vi "Create Virtual Drive.vi"(8 "error in (no error)":errorcluster, 11 "BuildWorker Controller in":refnum<class "BuildWorker Controller.lvclass">) -> (0 "error out":errorcluster, 3 "BuildWorker Controller out":refnum<class "BuildWorker Controller.lvclass">)   [LabVIEW 2017, in "BuildWorker Controller.lvlib" / "BuildWorker Controller.lvclass"]
uses:
  BuildWorker Controller.lvclass
  BuildWorker Controller.lvclass/BuildWorker Controller.ctl
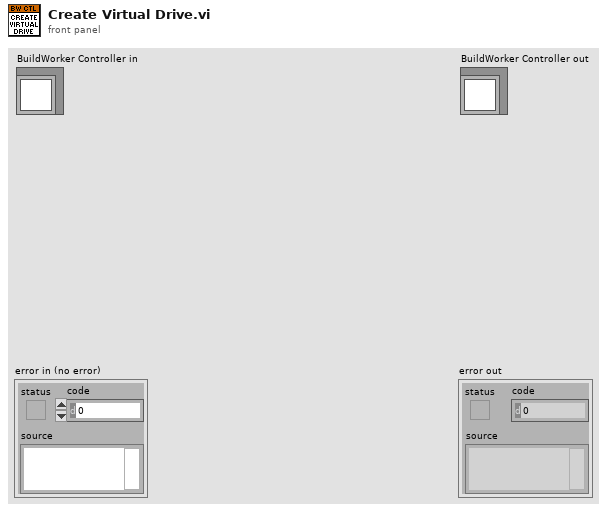
[diagram p1: front panel]
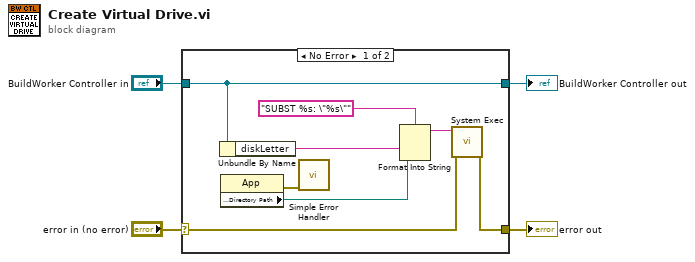
[diagram p0: block diagram]
diagram:
  n1 = case shown="No Error" "error in (no error)" {
    selector: "error in (no error)" -> [w7 w14]
    tunnel: [w6 w14] -> w3
    tunnel: [w12 w13] -> w1
    tunnel: "BuildWorker Controller in" -> [w12 w13]
    frame No Error {
      n2 = Unbundle By Name(w12) -> ("diskLetter"=w11:string)
      n3 = property class="App"() -> (error out=w10:errorcluster, "Application:Directory Path"=w5:path)  [unwired: 2 in, 1 out]
      n4 = call <vilib>:"Simple Error Handler.vi"("error in (no error)"=w10) -> ()  [unwired: 1 in, 8 out]
      n5 = Format Into String(format string="SUBST %s: \"%s\"", w11, w5) -> (resulting string=w8:string)  [unwired: 2 in, 1 out]
      n6 = call <vilib>:"System Exec.vi"("error in (no error)"=w7, "command line"=w8) -> ("error out"=w6:errorcluster)  [unwired: 6 in, 3 out]
    }
    frame Error {
    }
  }
  "error out" <- w3
  "BuildWorker Controller out" <- w1
